vi "Create default LV Icon Data.vi"(6 "New VI template? (F)":bool, 7 "Body Text":T1 {"Body Text Spec"."Alignment" items=["left", "center", "right"]}, 8 "error in":errorcluster, 11 "Pic Data in":T5) -> (0 "error out":errorcluster, 2 "VI Icon Data out":T4={"Text Visible?"=FALSE, "Text Opacity"=0, "Templ Visible?"=FALSE, "Templ Opacity"=0, "Relative Path from 1 to 2"=path "", "Image"=bytes[0], "All User Layers"=[], "Body Text"={"Line 1 text"="", "Line 2 text"="", "Line 3 text"="", "Line 4 text"="", "Line 1 color"=0, "Line 2 color"=0, "Line 3 color"=0, "Line 4 color"=0, "Body Text Spec"={"Font"="", "Alignment"=0, "Size"=3}, "Center text vertically"=FALSE, "Capitalize Text"=FALSE}} {"Body Text"."Body Text Spec"."Alignment" items=["left", "center", "right"]})   [LabVIEW 2012, in "lv_icon.lvlib"]
doc: "Populate the default LabVIEW Icon Data Cluster."
uses:
  <vilib>/LabVIEW Icon API/lv_icon/lv_icon.lvlib
  <vilib>/LabVIEW Icon API/lv_icon/Controls/LabVIEW Icon Stored Information.ctl
  <vilib>/LabVIEW Icon API/lv_icon/Classes/Layer/Layer.lvclass
  <vilib>/LabVIEW Icon API/lv_icon/Controls/BodyText.ctl
  <vilib>/LabVIEW Icon API/lv_icon/Controls/Font.ctl
  <vilib>/LabVIEW Icon API/lv_icon/Controls/Alignment.ctl
  <vilib>/LabVIEW Icon API/lv_icon/Controls/Layer.ctl
  <vilib>/LabVIEW Icon API/lv_icon/Controls/LayerType.ctl
panel:
  in  "LayerName":string="VI Icon"
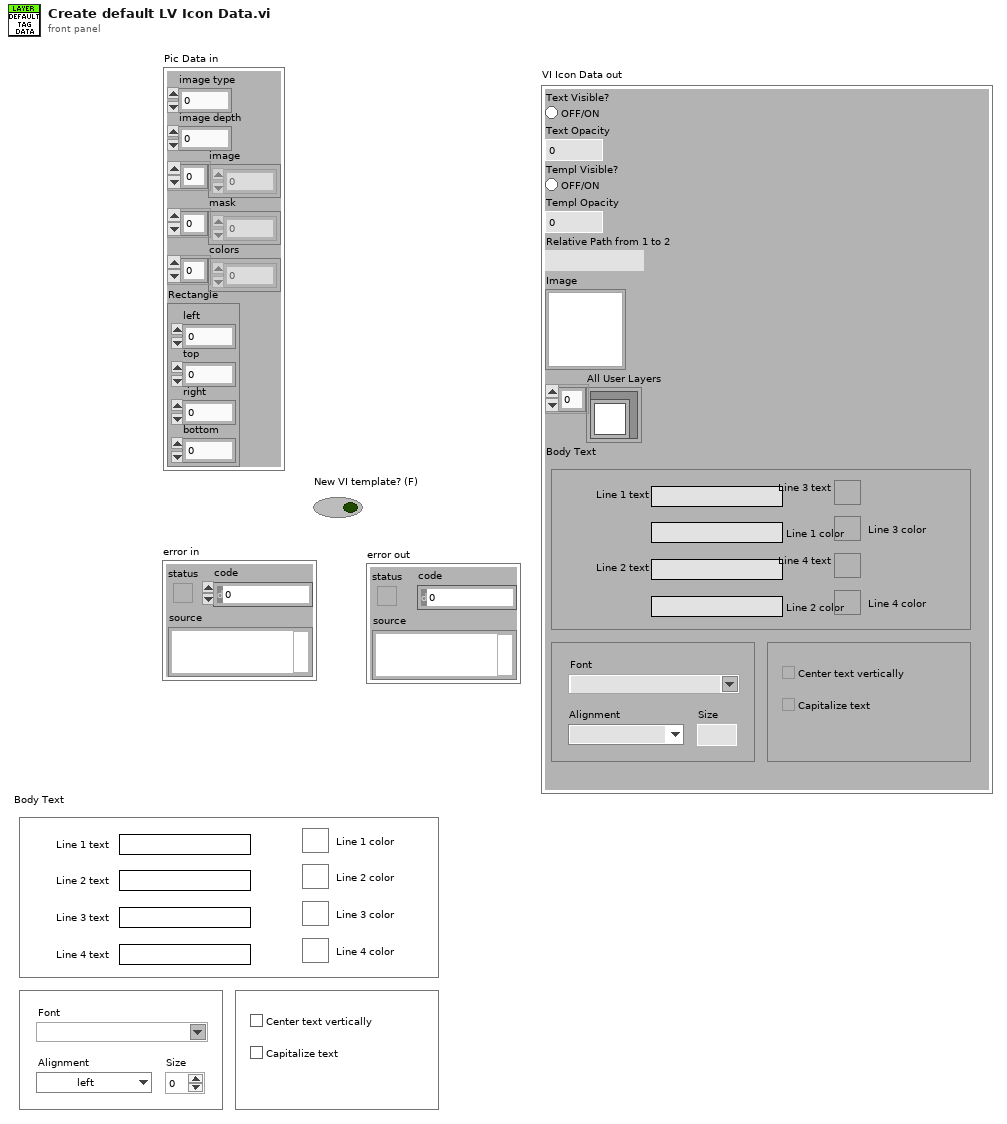
[diagram p1: front panel]
types:
  T1 = typedef "BodyText.ctl" = cluster{"Line 1 text":string, "Line 2 text":string, "Line 3 text":string, "Line 4 text":string, "Line 1 color":u32, "Line 2 color":u32, "Line 3 color":u32, "Line 4 color":u32, "Body Text Spec":cluster{"Font":T2, "Alignment":T3, "Size":u8}, "Center text vertically":bool, "Capitalize Text":bool}
  T2 = typedef "Font.ctl" = string
  T3 = typedef "Alignment.ctl" = u16
  T4 = typedef "LabVIEW Icon Stored Information.ctl" = cluster{"Text Visible?":bool, "Text Opacity":u8, "Templ Visible?":bool, "Templ Opacity":u8, "Relative Path from 1 to 2":path, "Image":picture, "All User Layers":refnum<class "Layer.lvclass">[], "Body Text":T1}
  T5 = cluster{"image type":i32, "image depth":i32, "image":u8[], "mask":u8[], "colors":u32[], "Rectangle":cluster{"left":i16, "top":i16, "right":i16, "bottom":i16}}
  T6 = typedef "LayerType.ctl" = enum16{"Graphic", "Text", "Tool", "Graphic Drop"}
  T7 = typedef "Layer.ctl" = cluster{"LayerIcon":picture, "LayerName":string, "Opacity":u8, "Visibility?":bool}
  T8 = typedef "imagedata.ctl" = cluster{"image type":i32, "image depth":i32, "image":u8[], "mask":u8[], "colors":u32[], "Rectangle":cluster{"left":i16, "top":i16, "right":i16, "bottom":i16}}
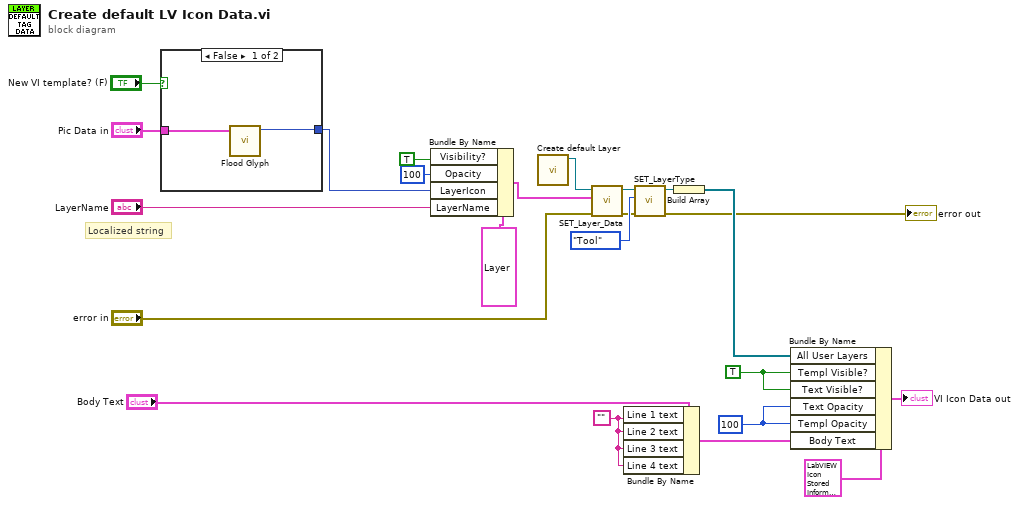
[diagram p0: block diagram]
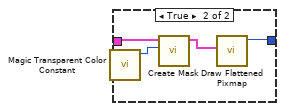
[diagram p2: hidden frame]
diagram:
  w10 = ""
  w8 = u8 100 ("Opacity")
  w7 = TRUE ("Visible?")
  # "Localized string"
  n1 = case shown="False" "New VI template? (F)" {
    tunnel: "Pic Data in" -> [w25 w28]
    tunnel: [w24 w27] -> w4
    frame False {
      n2 = call <vilib>:"Flood Glyph.vi"("image data"=w25) -> ("Pic Out"=w24:picture)  [unwired: 10 out]
    }
    frame True {
      n3 = call <vilib>:"Magic Transparent Color Constant.vi"() -> ("Magic transparent color constant"=w26:u32)  [unwired: 11 out]
      n4 = call <vilib>:"Create Mask.vi"("Mask Color (Black)"=w26, "image data"=w28) -> ("image data"=w29:T8)  [unwired: 9 in]
      n5 = call <vilib>:"Draw Flattened Pixmap.vi"("image data"=w29) -> ("new picture"=w27:picture)  [unwired: 8 in]
    }
  }
  n6 = Bundle By Name(cluster=T7 {"LayerIcon"=bytes[0], "LayerName"="", "Opacity"=0, "Visibility?"=FALSE} ("Data"), "Visibility?"=TRUE, "Opacity"=u8 100, "LayerIcon"=w4, "LayerName"="LayerName") -> (w18:T7)
  n7 = call <vilib>:"Create default Layer.vi"() -> ("Layer.lvclass out"=w3:refnum<class "Layer.lvclass">)  [unwired: 1 in, 10 out]
  n8 = call-dynamic "SET_Layer_Data.vi"("error in (no error)"="error in", "Data"=w18, "Layer.lvclass in"=w3) -> ("error out"=w14:errorcluster, "Layer.lvclass out"=w19:refnum<class "Layer.lvclass">)  [unwired: 1 in, 6 out]
  n9 = Bundle By Name(cluster="Body Text", "Line 1 text"=w10, "Line 2 text"=w10, "Line 3 text"=w10, "Line 4 text"=w10) -> (w9:T1)
  n10 = call-dynamic "SET_LayerType.vi"("error in (no error)"=w14, "Type"=LayerType."Tool", "Layer.lvclass in"=w19) -> ("error out"=→"error out":errorcluster, "Layer.lvclass out"=w20:refnum<class "Layer.lvclass">)  [unwired: 7 out]
  n11 = Build Array(w20) -> (w15:refnum<class "Layer.lvclass">[])
  n12 = Bundle By Name(cluster=T4 {"Text Visible?"=FALSE, "Text Opacity"=0, "Templ Visible?"=FALSE, "Templ Opacity"=0, "Relative Path from 1 to 2"=path "", "Image"=bytes[0], "All User Layers"=[], "Body Text"={"Line 1 text"="", "Line 2 text"="", "Line 3 text"="", "Line 4 text"="", "Line 1 color"=0, "Line 2 color"=0, "Line 3 color"=0, "Line 4 color"=0, "Body Text Spec"={"Font"="", "Alignment"=0, "Size"=3}, "Center text vertically"=FALSE, "Capitalize Text"=FALSE}} ("VI Icon Data in"), "All User Layers"=w15, "Templ Visible?"=w7, "Text Visible?"=w7, "Text Opacity"=w8, "Templ Opacity"=w8, "Body Text"=w9) -> (→"VI Icon Data out":T4)
